vi "Handle Error.vi"(8 "error in (no error)":errorcluster, 11 "XY Stage Process in":refnum<class "XY Stage Process.lvclass">) -> (0 "error out":errorcluster, 2 "stop actor?":bool=TRUE, 3 "XY Stage Process out":refnum<class "XY Stage Process.lvclass">)   [LabVIEW 2022 SP3, in "XY Stage Process.lvlib" / "XY Stage Process.lvclass"]
doc: "(<B>Filename</B>: Actor Framework.lvlib:Actor.lvclass:Handle Error.vi)\n\nDefines how the actor handles an error that occurred while processing a message.\n\nBy default, this method does nothing except stop the actor. This method also treats error code 43 (coming from <B>error in</B>) as a sign that the actor shut down normally. In this situation, the Handle Error method does not return the error on <B>error out</B>, meaning the actor's caller will not receive it. All other error codes will be returned on <B>error out</B>.\n\nA descendant class may override this method to change this behavior."
uses:
  XY Stage Process.lvclass
  XY Stage Process.lvclass/XY Stage Process.ctl
  Process Framework/Process State Data/Process State Data.lvclass
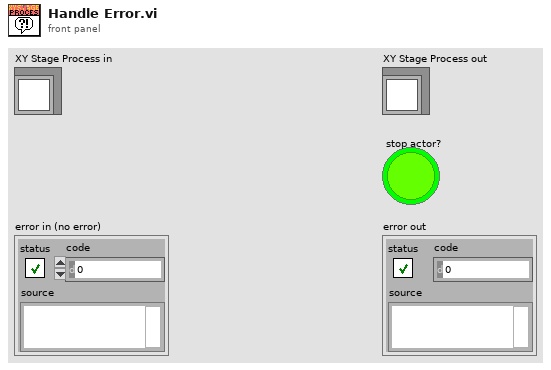
[diagram p1: front panel]
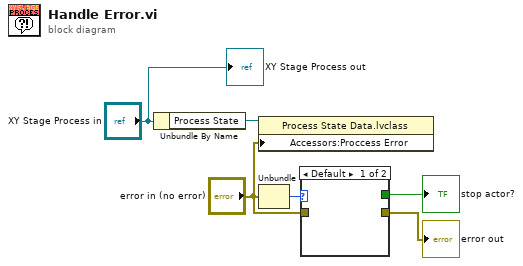
[diagram p0: block diagram]
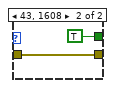
[diagram p2: hidden frame]
diagram:
  n1 = Unbundle By Name("XY Stage Process in") -> ("Process State"=w2:refnum<data-value>)
  n2 = property class="Process State Data.lvclass"(reference=w2, "Accessors:Proccess Error"="error in (no error)") -> ()  [unwired: 1 in, 2 out]
  n3 = Unbundle("error in (no error)") -> ("code"=w5:i32)  [unwired: 2 out]
  n4 = case shown="Default" w5 {
    tunnel: [_ w7] -> w6
    tunnel: "error in (no error)" -> [_ w7]
    tunnel: [_ TRUE] -> w4
    frame Default {
    }
    frame 43, 1608 {
    }
  }
  "error out" <- w6
  "stop actor?" <- w4
  "XY Stage Process out" <- "XY Stage Process in"
